vi "post math 3(SubVI).vi"() -> ()   [LabVIEW 2020]
panel:
  in  "raw magnatude":dbl
  in  "x":dbl
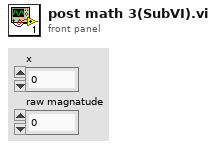
[diagram p1: front panel]
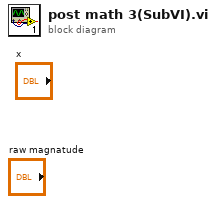
[diagram p0: block diagram]
diagram:
